vi "FindData.vi"(2 "Value In":string, 3 "Item":string="Data", 4 "Data In":string[][](table)) -> (0 "Value Out":string, 1 "Data Out":string[][](table))   [LabVIEW 2014]
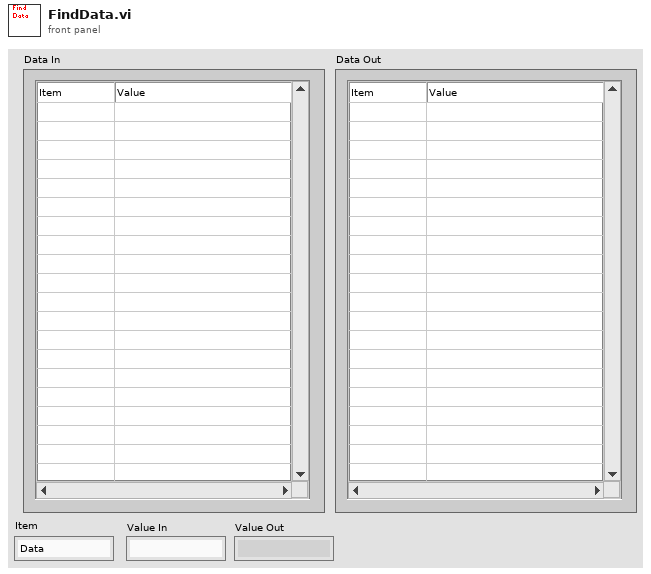
[diagram p1: front panel]
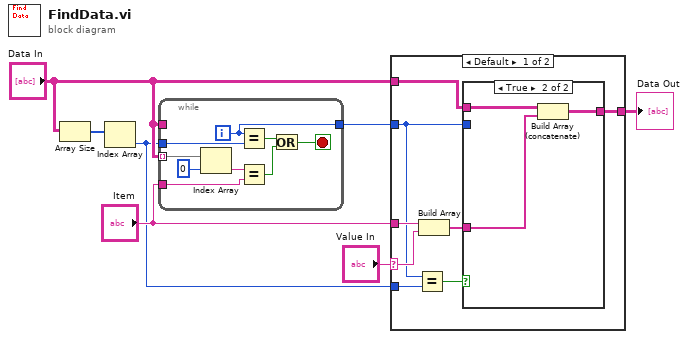
[diagram p0: block diagram]
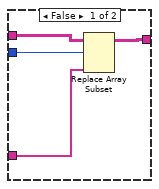
[diagram p2: hidden frame]
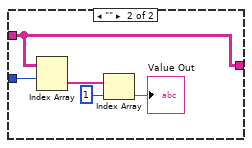
[diagram p3: hidden frame]
diagram:
  n1 = Array Size(array="Data In") -> (size(s)=w7:i32[])
  n2 = Index Array(array=w7) -> (element=w2:i32)  [unwired: 1 in]
  n3 = while {
    tunnel: "Data In" -> [w16] mode=indexing
    tunnel: [w8] -> w1
    tunnel: w2 -> [w13]
    tunnel: "Data In" -> [_]
    tunnel: "Item" -> [w9]
    i -> [w8]
    stop <- w12 stop-if-true
    n4 = Index Array(array=w16, index=0) -> (element=w11:string)
    n5 = Equal?(x=w8, y=w13) -> (x = y?=w14:bool)
    n6 = Equal?(x=w11, y=w9) -> (x = y?=w10:bool)
    n7 = Or(x=w14, y=w10) -> (x .or. y?=w12:bool)
  }
  n8 = case shown="Default" "Value In" {
    selector: "Value In" -> [w24 _]
    tunnel: [w22 w33] -> w6
    tunnel: "Data In" -> [w21 w33]
    tunnel: w1 -> [w19 w32]
    tunnel: "Item" -> [w20 _]
    tunnel: w2 -> [w18 _]
    frame Default {
      n9 = Equal?(x=w19, y=w18) -> (x = y?=w17:bool)
      n10 = Build Array(w20, w24) -> (w23:string[])
      n11 = case shown="True" w17 {
        tunnel: w23 -> [w28 w30]
        tunnel: [w27 w29] -> w22
        tunnel: w21 -> [w26 w31]
        tunnel: w19 -> [w25 _]
        frame False {
          n12 = Replace Array Subset(array=w26, new element=w28, index (row)=w25) -> (w27:string[][])  [unwired: 1 in]
        }
        frame True {
          n13 = Build Array (concatenate)(w31, w30) -> (w29:string[][])
        }
      }
    }
    frame "" {
      n14 = Index Array(array=w33, index (row)=w32) -> (element=w35:string[])  [unwired: 1 in]
      n15 = Index Array(array=w35, index=1) -> (element=→"Value Out":string)
    }
  }
  "Data Out" <- w6
